vi "ReadTemp.vi"(0 "COMPORT":refnum<visa-resource-name>="COM1", 1 "#ofAvgs":i32=1 min=1 max=9999 step=1, 5 "ILabVIEW":refnum<k24>, 11 "Error In":errorcluster, 12 "InstanceId":i32=1, 13 "close session(t)":bool=TRUE, 14 "OpenSession(t)":bool) -> (3 "Deg":dbl format="%.3g", 4 "comport":refnum<visa-resource-name>="COM1", 6 "ILabVIEW Out":refnum<k24>, 15 "error out":errorcluster)   [LabVIEW 2018]
uses:
  C:/RageATE/Instruments/Ess Temp Plate/LabView Driver/Public/Watbus.dll
  LabView Driver/Public/Watbus.dll
  <vilib>/Analysis/baseanly.llb/Mean (DBL).vi
  <vilib>/Analysis/NI_AALBase.lvlib
panel:
  out "Value Out":string
  in  "TemperatureUnits":u8(ring)=1 items=["Degrees F", "Degrees C"]
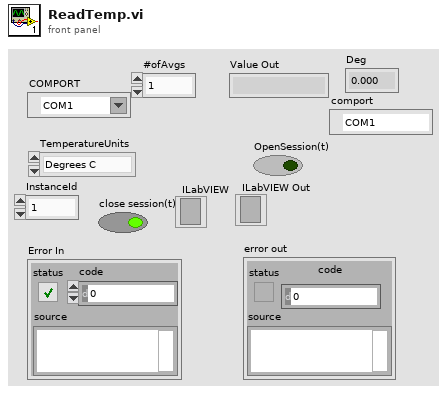
[diagram p1: front panel]
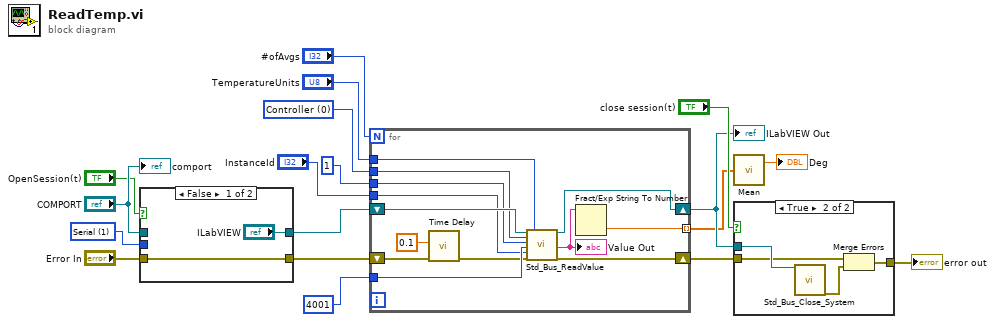
[diagram p0: block diagram]
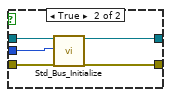
[diagram p2: hidden frame]
diagram:
  w13 = 1 items=["Usb", "Serial", "Ethernet", "Unconnected"] ("InterfaceType")
  w15 = 0 items=["Controller", "RUI", "PC", "CommsCard"] ("deviceType")
  n1 = case shown="False" "OpenSession(t)" {
    tunnel: "COMPORT" -> [_ w25]
    tunnel: w13 -> [_ w24]
    tunnel: "Error In" -> [w20 w23]
    tunnel: ["ILabVIEW" w22] -> w6
    tunnel: [w20 w21] -> w5
    frame False {
    }
    frame True {
      n2 = call "Std_Bus_Initialize.vi"("Communications Port"=w25, "InterfaceType"=w24, "error in (no error)"=w23) -> ("ILabVIEW"=w22:refnum<k24>, "error out"=w21:errorcluster)  [unwired: 14 in, 1 out]
    }
  }
  n3 = for {
    N: "#ofAvgs" -> [_]
    tunnel: w15 -> [w35]
    tunnel: 4001 ("ParameterID") -> [w34]
    tunnel: "InstanceId" -> [w33]
    tunnel: 1 ("Zone") -> [w32]
    tunnel: "TemperatureUnits" -> [w31]
    shift-right: [w36] -> w16
    shift-left: w6 -> [w38]
    shift-right: [w30] -> w10
    shift-left: w5 -> [w37]
    tunnel: [w28] -> w3 mode=indexing
    n4 = call "Time Delay"("error in (no error)"=w37, "Delay Time (s)"=0.1) -> ("error out"=w26:errorcluster)  [unwired: 9 in]
    n5 = call "Std_Bus_ReadValue.vi"("ILabVIEW In"=w38, "DeviceType"=w35, "Zone"=w32, "ParameterID"=w34, "InstanceId"=w33, "error in (no error)"=w26, "TemperatureUnits"=w31) -> ("ILabVIEW Out"=w36:refnum<k24>, "Value Out"=w29:string, "error out"=w30:errorcluster)  [unwired: 10 in]
    "Value Out" <- w29
    n6 = Fract/Exp String To Number(string=w29) -> (number=w28:dbl)  [unwired: 3 in, 1 out]
  }
  "ILabVIEW Out" <- w16
  n7 = call-poly <vilib>:"Mean.vi"("X"=w3) -> ("mean"=→"Deg":dbl)  [unwired: 1 out]
  n8 = case shown="True" "close session(t)" {
    tunnel: w16 -> [_ w43]
    tunnel: [w39 w40] -> w11
    tunnel: w10 -> [w39 w42]
    frame False {
    }
    frame True {
      n9 = call "Std_Bus_Close_System.vi"("ILabVIEW In"=w43) -> ("error out"=w41:errorcluster)  [unwired: 18 in]
      n10 = Merge Errors(w42, w41) -> (w40:errorcluster)
    }
  }
  "error out" <- w11
  "comport" <- "COMPORT"
